vi "Get-priority-message.vi"(8 "error in (no error)":errorcluster, 9 "Additional content":string, 10 "Priority message":T1) -> (0 "error out":errorcluster, 2 "Message string":string)   [LabVIEW 2013, in "HardwareCharacterization.lvlib" / "HC-SM1000.lvclass"]
uses:
  HC-SM1000.lvclass
  Priority-messages.ctl
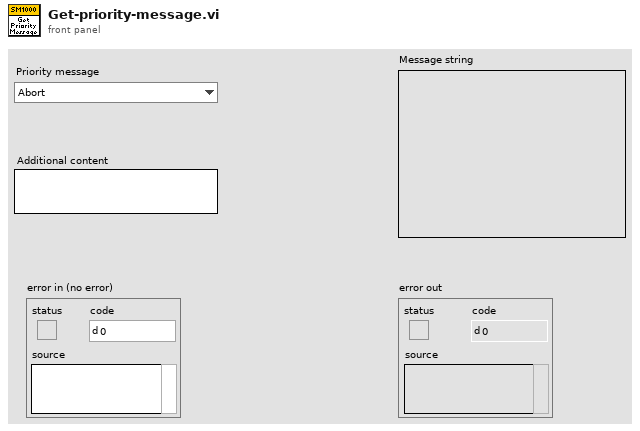
[diagram p1: front panel]
types:
  T1 = typedef "HardwareCharacterization.lvlib/HC-SM1000.lvclass/Priority-messages.ctl" = enum16{"Abort", "Restart", "Suspend", "Resume", "GetRegisters", "SetInterlockEnable", "SetOffset"}
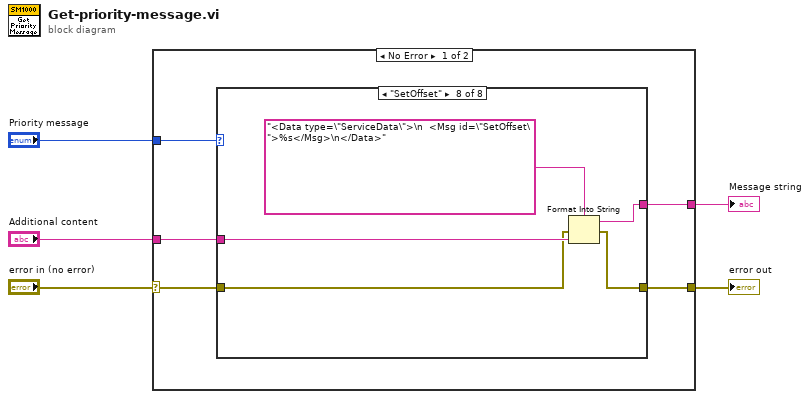
[diagram p0: block diagram]
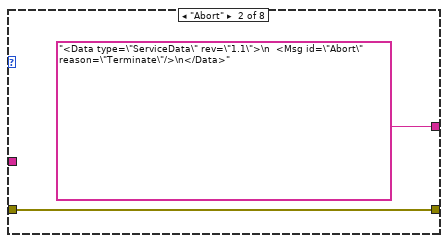
[diagram p3: hidden frame]
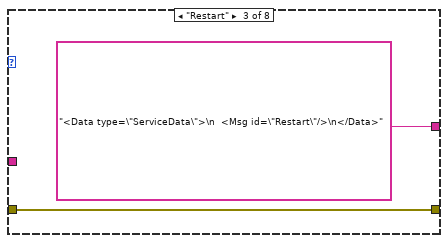
[diagram p4: hidden frame]
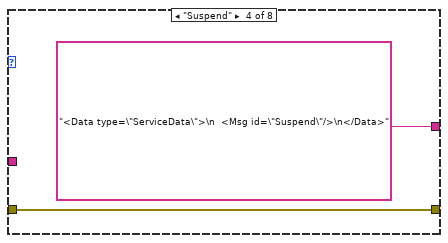
[diagram p5: hidden frame]
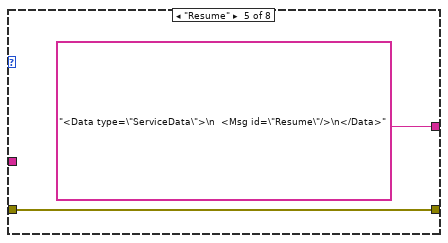
[diagram p6: hidden frame]
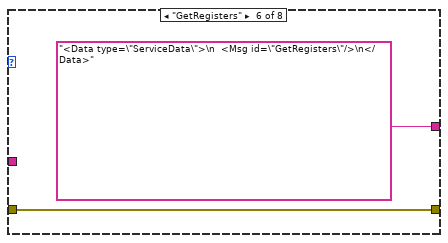
[diagram p7: hidden frame]
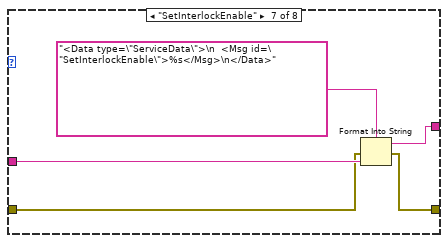
[diagram p8: hidden frame]
diagram:
  n1 = case shown="No Error" "error in (no error)" {
    selector: "error in (no error)" -> [w9 w32]
    tunnel: [w8 w32] -> w4
    tunnel: "Priority message" -> [w10 _]
    tunnel: [w7 _] -> w2
    tunnel: "Additional content" -> [w6 _]
    frame No Error {
      n2 = case shown="\"SetOffset\"" w10 {
        tunnel: w9 -> [w11 w13 w15 w17 w19 w21 w23 w28]
        tunnel: [w11 w13 w15 w17 w19 w21 w22 w27] -> w8
        tunnel: [_ "<Data type=\"ServiceData\" rev=\"1.1\">\n  <Msg id=\"Abort\" reason=\"Terminate\"/>\n</Data>" "<Data type=\"ServiceData\">\n  <Msg id=\"Restart\"/>\n</Data>" "<Data type=\"ServiceData\">\n  <Msg id=\"Suspend\"/>\n</Data>" "<Data type=\"ServiceData\">\n  <Msg id=\"Resume\"/>\n</Data>" "<Data type=\"ServiceData\">\n  <Msg id=\"GetRegisters\"/>\n</Data>" w25 w30] -> w7
        tunnel: w6 -> [_ _ _ _ _ _ w24 w29]
        frame Default {
        }
        frame "Abort" {
        }
        frame "Restart" {
        }
        frame "Suspend" {
        }
        frame "Resume" {
        }
        frame "GetRegisters" {
        }
        frame "SetInterlockEnable" {
          n3 = Format Into String(format string="<Data type=\"ServiceData\">\n  <Msg id=\"SetInterlockEnable\">%s</Msg>\n</Data>", error in=w23, w24) -> (resulting string=w25:string, error out=w22:errorcluster)  [unwired: 1 in]
        }
        frame "SetOffset" {
          n4 = Format Into String(format string="<Data type=\"ServiceData\">\n  <Msg id=\"SetOffset\">%s</Msg>\n</Data>", error in=w28, w29) -> (resulting string=w30:string, error out=w27:errorcluster)  [unwired: 1 in]
        }
      }
    }
    frame Error {
    }
  }
  "error out" <- w4
  "Message string" <- w2
